vi "1A TemperatureLogger.vi"() -> ()   [LabVIEW 2011]
uses:
  <vilib>/Platform/storage/Storage.llb/usiOverwriteOptions.ctl
  <vilib>/Platform/storage/Storage.llb/usiSequenceRepresentation.ctl
  <vilib>/FPGAPlugInAG/cRIO-9113/niLvFpga_Open_cRIO-9113.vi
  <vilib>/rvi/interface/common/dynamic/niFpgaDynamicAddResources.vi
  <vilib>/Utility/error.llb/Error Cluster From Error Code.vi
  <vilib>/rvi/errors/niLvFpgaAdjustHostInterfaceError.vi
  <vilib>/FPGAPlugInAG/Dynamic/niLvFpga_Close_Dynamic.vi
  <vilib>/Platform/storage/lvStorage.llb/_defaultFilePath.vi
  <vilib>/Platform/storage/lvStorage.llb/_openStorageWithRootAutoDetect.vi
  <vilib>/Platform/storage/lvStorage.llb/xStorage/xStorageSupp/ErrorOut.vi
  <vilib>/Platform/storage/lvStorage.llb/_createOrGetExplicitChildObject.vi
  <vilib>/Platform/storage/lvStorage.llb/_createOrGetByNameExplicitChildObject.vi
  <vilib>/Platform/storage/lvStorage.llb/_saveInt16Channel.vi
  <vilib>/Platform/storage/Storage.llb/Get Object Info.vi
  <vilib>/Platform/storage/Storage.llb/__closeStorageFromObject.vi
  <vilib>/rvi/interface/nirviOpenFPGA/nirviOpenFPGA.xnode
  FPGA Bitfiles/SailBot_FPGATarget_1ATemperatureRea_2D2CF993.lvbitx
  FPGA/1A Temperature Reader.vi
  <vilib>/rvi/interface/nirviMethod/nirviMethod.xnode
  <vilib>/rvi/interface/nirviCloseFPGA/nirviCloseFPGA.xnode
  <vilib>/Platform/storage/lvStorage.llb/xStorage/Open Data Storage/Open Data Storage.xnode
  <vilib>/Platform/storage/lvStorage.llb/xStorage/Write Data/Write Data.xnode
  <vilib>/Platform/storage/lvStorage.llb/xStorage/Close Data Storage/Close Data Storage.xnode
  <vilib>/FPGAPlugInAG/Dynamic/niLvFpga_ReadFifo_Dynamic.vi
  <vilib>/rvi/errors/niLvFpgaMergeErrorWithErrorCode.vi
panel:
  out "Default Directory":path
  out "Temperature Data":i16[](graph)
  in  "stop":bool
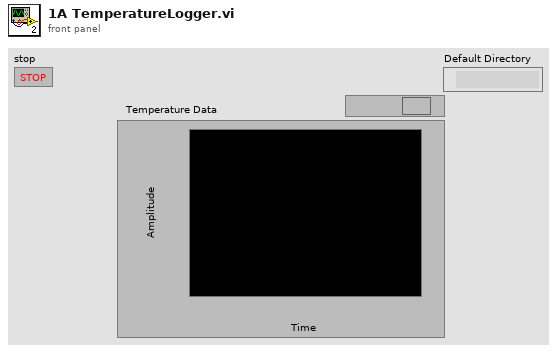
[diagram p1: front panel]
types:
  T1 = enum16{"open", "open or create", "create or replace", "create", "open (read only)"}
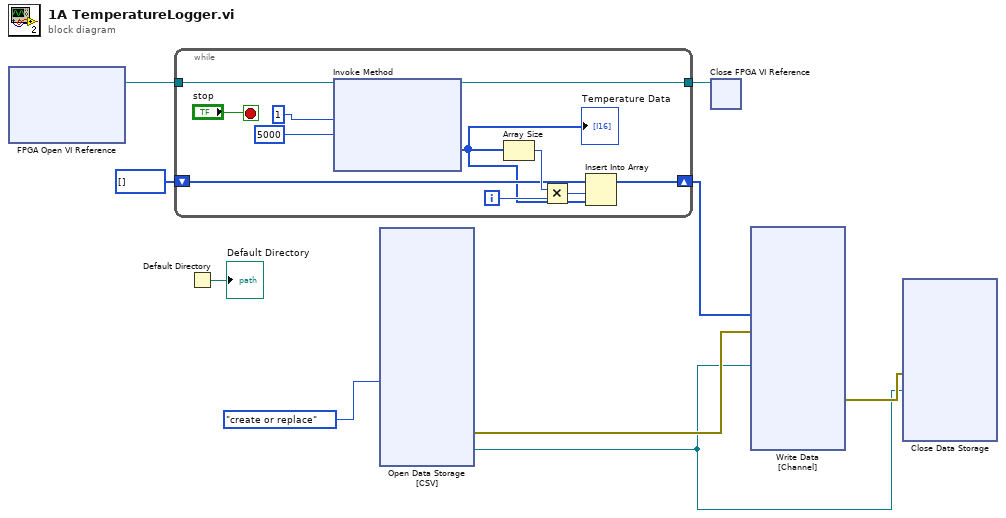
[diagram p0: block diagram]
diagram:
  n1 = xnode "FPGA Open VI Reference"() -> ("FPGA VI Reference Out"=w6:refnum<k20>)  [unwired: 2 in, 1 out]
  n2 = while {
    tunnel: w6 -> [w19]
    tunnel: [w18] -> w7
    shift-right: [w17] -> w4
    shift-left: i16[] [] -> [w13]
    i -> [w14]
    stop <- "stop" stop-if-true
    n3 = xnode "Invoke Method"("FPGA VI Reference In"=w19, "Number of Elements"=u32 1, "Timeout (ms)"=5000) -> ("FPGA VI Reference Out"=w18:refnum<k20>, "Data"=w10:i16[])  [unwired: 1 in, 2 out]
    "Temperature Data" <- w10
    n4 = Array Size(array=w10) -> (size(s)=w15:i32)
    n5 = Multiply(x=w15, y=w14) -> (x*y=w16:i32)
    n6 = Insert Into Array(array=w13, index=w16, new element=w10) -> (w17:i16[])
  }
  n7 = Default Directory() -> (→"Default Directory":path)
  n8 = xnode "Open Data Storage\n[CSV]"("function (open:0)"=T1."create or replace") -> ("error out"=w9:errorcluster, "storage refnum (file)"=w1:refnum<k20>)  [unwired: 4 in, 1 out]
  n9 = xnode "Close FPGA VI Reference"("FPGA VI Reference In"=w7) -> ()  [unwired: 1 in, 1 out]
  n10 = xnode "Write Data\n[Channel]"("Signal"=w4, "error in"=w9, "storage refnum (file)"=w1) -> ("error out"=w8:errorcluster)  [unwired: 2 in, 2 out]
  n11 = xnode "Close Data Storage\n"("error in (no error)"=w8, "storage refnum (file)"=w1) -> ()  [unwired: 2 out]
